vi "plc传输点位补偿.vi"(8 "选项":enum16{"布线前甩线", "布线", "布线后甩线"}(ring), 9 "基本信息":T1, 10 "行":i32, 11 "数组输入":dbl[](array[numeric])) -> (3 "数组输出":dbl[](array[numeric]))   [LabVIEW 2014]
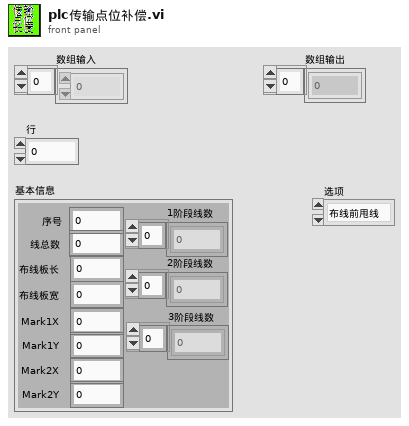
[diagram p1: front panel]
types:
  T1 = typedef "基本信息.ctl" = cluster{"序号":dbl, "线总数":dbl, "布线板长":dbl, "布线板宽":dbl, "Mark1X":dbl, "Mark1Y":dbl, "Mark2X":dbl, "Mark2Y":dbl, "1阶段线数":dbl[], "2阶段线数":dbl[], "3阶段线数":dbl[]}
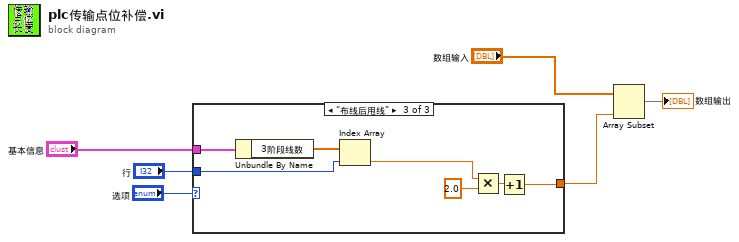
[diagram p0: block diagram]
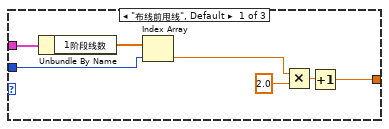
[diagram p2: hidden frame]
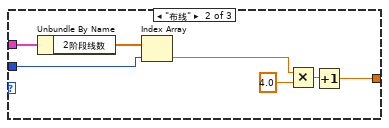
[diagram p3: hidden frame]
diagram:
  n1 = case shown="\"布线后甩线\"" "选项" {
    tunnel: [w11 w20 w25] -> w6
    tunnel: "基本信息" -> [w9 w16 w23]
    tunnel: "行" -> [w7 w14 w22]
    frame "布线前甩线", Default {
      n2 = Unbundle By Name(w9) -> ("1阶段线数"=w10:dbl[])
      n3 = Index Array(array=w10, index=w7) -> (element=w8:dbl)
      n4 = Multiply(x=w8, y=2.0) -> (x*y=w13:dbl)
      n5 = Increment(x=w13) -> (x+1=w11:dbl)
    }
    frame "布线" {
      n6 = Unbundle By Name(w16) -> ("2阶段线数"=w15:dbl[])
      n7 = Index Array(array=w15, index=w14) -> (element=w17:dbl)
      n8 = Multiply(x=w17, y=4.0) -> (x*y=w19:dbl)
      n9 = Increment(x=w19) -> (x+1=w20:dbl)
    }
    frame "布线后甩线" {
      n10 = Unbundle By Name(w23) -> ("3阶段线数"=w24:dbl[])
      n11 = Index Array(array=w24, index=w22) -> (element=w21:dbl)
      n12 = Multiply(x=w21, y=2.0) -> (x*y=w27:dbl)
      n13 = Increment(x=w27) -> (x+1=w25:dbl)
    }
  }
  n14 = Array Subset(array="数组输入", length=w6) -> (→"数组输出":dbl[])  [unwired: 1 in]
